vi "Finalize To Settings.vi"(8 "error in":errorcluster, 11 "RDMA Tx Transfer Configuration in":refnum<class "RDMA Transfer Tx Configuration.lvclass">) -> (0 "error out":errorcluster, 2 "settings":cluster{"key":string, "value":string}[](array[cluster]), 3 "RDMA Tx Transfer Configuration out":refnum<class "RDMA Transfer Tx Configuration.lvclass">)   [LabVIEW 2020, in "RDMA.lvlib" / "RDMA Transfer Tx Configuration.lvclass"]
uses:
  RDMA Transfer Tx Configuration.lvclass
  RDMA Transfer Tx Configuration.lvclass/RDMA Transfer Tx Configuration.ctl
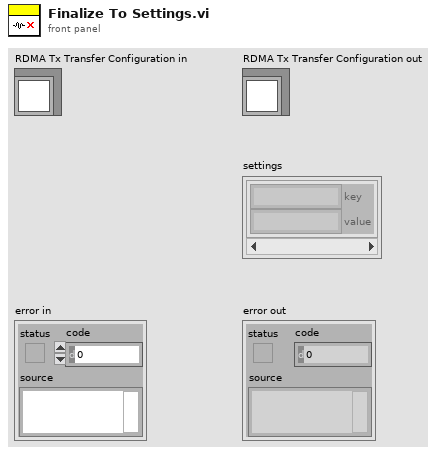
[diagram p1: front panel]
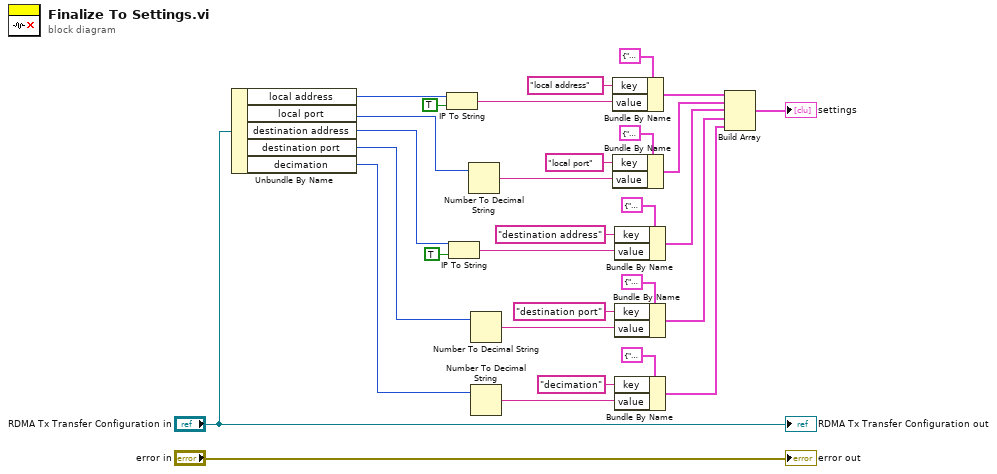
[diagram p0: block diagram]
diagram:
  n1 = Unbundle By Name("RDMA Tx Transfer Configuration in") -> ("local address"=w27:u32, "local port"=w22:u16, "destination address"=w13:u32, "destination port"=w12:u16, "decimation"=w2:u16)
  n2 = IP To String(1:TRUE ("dot notation? (F)"), 2:w27) -> (0:w25:string)
  n3 = IP To String(1:TRUE ("dot notation? (F)"), 2:w13) -> (0:w17:string)
  n4 = Number To Decimal String(number=w22) -> (decimal integer string=w21:string)  [unwired: 1 in]
  n5 = Number To Decimal String(number=w12) -> (decimal integer string=w20:string)  [unwired: 1 in]
  n6 = Number To Decimal String(number=w2) -> (decimal integer string=w5:string)  [unwired: 1 in]
  n7 = Bundle By Name(cluster=cluster{"key":string, "value":string} {"key"="", "value"=""} ("setting"), "key"="local address", "value"=w25) -> (w11:cluster{"key":string, "value":string})
  n8 = Bundle By Name(cluster=cluster{"key":string, "value":string} {"key"="", "value"=""} ("setting"), "key"="local port", "value"=w21) -> (w10:cluster{"key":string, "value":string})
  n9 = Bundle By Name(cluster=cluster{"key":string, "value":string} {"key"="", "value"=""} ("setting"), "key"="destination address", "value"=w17) -> (w9:cluster{"key":string, "value":string})
  n10 = Bundle By Name(cluster=cluster{"key":string, "value":string} {"key"="", "value"=""} ("setting"), "key"="destination port", "value"=w20) -> (w8:cluster{"key":string, "value":string})
  n11 = Bundle By Name(cluster=cluster{"key":string, "value":string} {"key"="", "value"=""} ("setting"), "key"="decimation", "value"=w5) -> (w1:cluster{"key":string, "value":string})
  n12 = Build Array(w11, w10, w9, w8, w1) -> (→"settings":cluster{"key":string, "value":string}[])
  "error out" <- "error in"
  "RDMA Tx Transfer Configuration out" <- "RDMA Tx Transfer Configuration in"
